vi "initializeArcus.vi"(1 "device_index (in) [0=def]":i32, 2 "read_timeout (ms); def=1000":i32=1000, 3 "write_timeout (ms); def=1000":i32=1000, 4 "clear_buffer? (T)":bool=TRUE, 5 "error in (no error)":errorcluster, 7 "error dialog? (T)":bool=TRUE) -> (14 "reference (out)":refnum<class "_Controller.lvclass">, 19 "error out":errorcluster)   [LabVIEW 2020, in "classes.lvlib" / "_Controller.lvclass"]
doc: "This VI establishes a reference to the USB Arcus controller at the specified index. Additionally, a LabVIEW based Class is instantiated, representing the specific device model. Additionally, parameters such as USB Reference, Index, Description, Name and other parameters are all set to the reference for ease of access downstream.\n\nOther inputs to be aware of:\n\n<B>device_index</B>: the index specific to the attached device (the index input is \"zero\" indexed - meaning the first of all devices sits at index = \"0\" and NOT \"1\")\n<B>read_timeout (ms)</B>: the USB \"read\" timeout in milliseconds (defaults to 1000ms)\n<B>write_timeout (ms)</B>: the USB \"write\" timeout in milliseconds (defaults to 1000ms)\n<B>clear_buffer?</B>: if set to TRUE, a USB Buffer CLEAR is issued (default is TRUE)\n<B>error_dialog?</B>: if set to TRUE, any errors triggered during USB controller communications result in a dialog window appearing at the moment the error is detected. If set to FALSE, the error is carried through via the error cluster. Default is TRUE.\n\nProduced By:\n\n<B>Kod Integrations, LLC</B>\n4835 Marianne Drive\nMount Airy, MD 21771\nhttp://www.kodintegrations.com\nemail: info@kodintegrations.com\nphone: (240) 687-1288"
uses:
  _Controller.lvclass
  DMXJSAController.lvclass
  Pmx4exSaController.lvclass
  ACESDEController.lvclass
  _SingleAxisController.lvclass
  PMX4CXSAController.lvclass
  PMX2EXSAController.lvclass
  C:/GEECS/Developers Version/source/Device Drivers/Newmark-NSC-A/Arcus Driver 3.0.0/ArcusUsbComm/classes/SingleAxisController/_SingleAxisController.lvclass
  C:/GEECS/Developers Version/source/Device Drivers/Newmark-NSC-A/Arcus Driver 3.0.0/ArcusUsbComm/classes/Controller/_Controller.lvclass
  C:/GEECS/Developers Version/source/Device Drivers/Newmark-NSC-A/Arcus Driver 3.0.0/ArcusUsbComm/classes/DMX-J-SA/DMXJSAController.lvclass
  C:/GEECS/Developers Version/source/Device Drivers/Newmark-NSC-A/Arcus Driver 3.0.0/ArcusUsbComm/classes/ACE-SDE/ACESDEController.lvclass
  C:/GEECS/Developers Version/source/Device Drivers/Newmark-NSC-A/Arcus Driver 3.0.0/ArcusUsbComm/classes/MultiAxisController/_MultiAxisController.lvclass
  C:/GEECS/Developers Version/source/Device Drivers/Newmark-NSC-A/Arcus Driver 3.0.0/ArcusUsbComm/classes/PMX-4EX-SA/Pmx4exSaController.lvclass
  C:/GEECS/Developers Version/source/Device Drivers/Newmark-NSC-A/Arcus Driver 3.0.0/ArcusUsbComm/classes/PMX-4CX-SA/PMX4CXSAController.lvclass
  C:/GEECS/Developers Version/source/Device Drivers/Newmark-NSC-A/Arcus Driver 3.0.0/ArcusUsbComm/classes/PMX-2EX-SA/PMX2EXSAController.lvclass
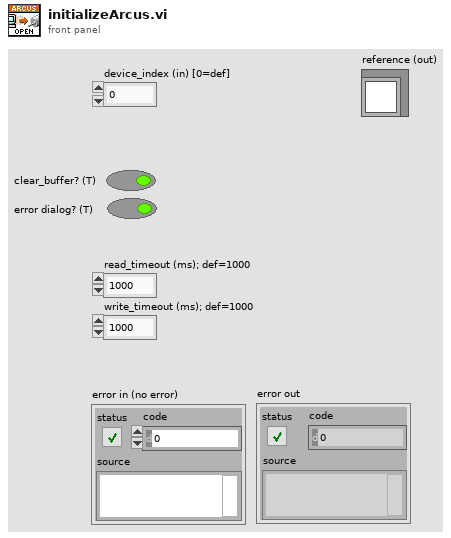
[diagram p1: front panel]
types:
  T1 = typedef "common.lvlib/device_info.ctl" = cluster{"device_name":string, "device_description":string, "model":T2}
  T2 = typedef "common.lvlib/models.ctl" = enum16{"<unrecognized>", "ACE-SDC", "ACE-SDE", "ACE-SXC", "ACE-SXE", "DMX-CAN", "DMX-J-SA", "DMX-K-SA", "DMX-UMD", "PMX-2ED-SA", "PMX-2EX-SA", "PMX-4CX-SA", "PMX-4EX-SA"}
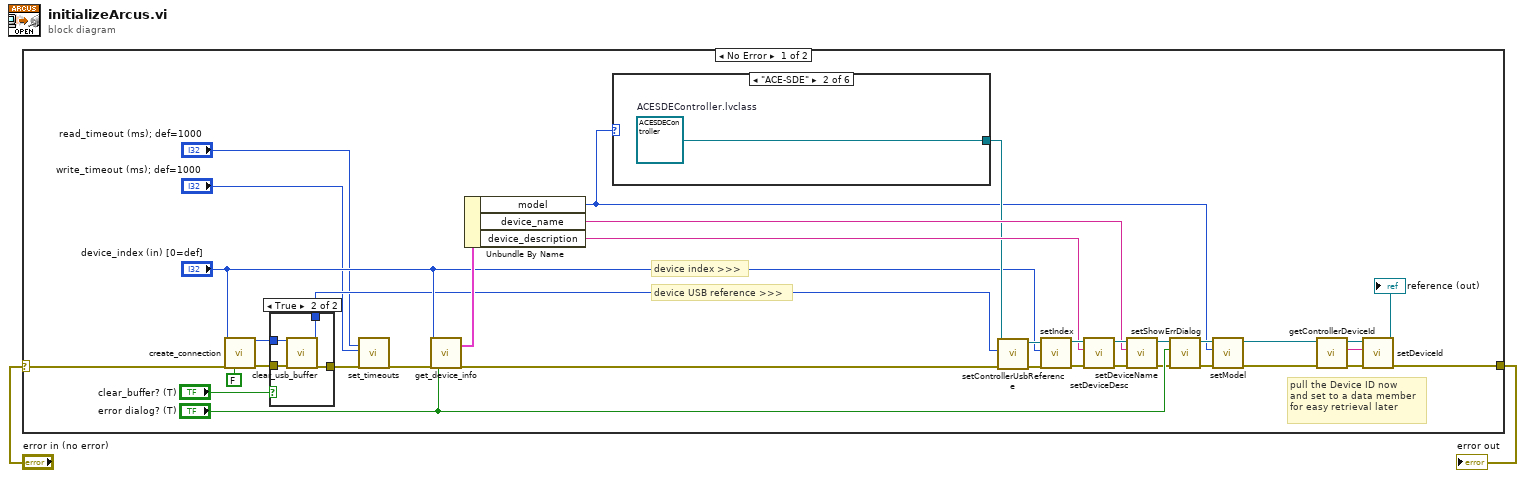
[diagram p0: block diagram]
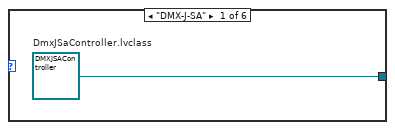
[diagram p3: hidden frame]
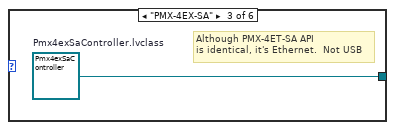
[diagram p4: hidden frame]
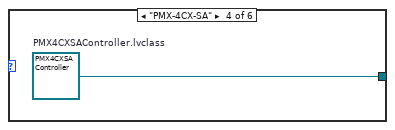
[diagram p5: hidden frame]
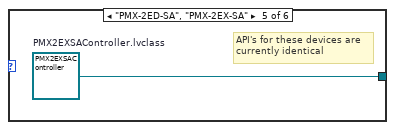
[diagram p6: hidden frame]
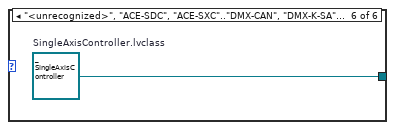
[diagram p7: hidden frame]
diagram:
  n1 = case shown="No Error" "error in (no error)" {
    selector: "error in (no error)" -> [w30 w50]
    tunnel: [w14 w50] -> w1
    frame No Error {
      # "device USB reference >>>"
      # "device index >>>"
      # "pull the Device ID now\nand set to a data member\nfor easy retrieval later"
      n2 = call "create_connection.vi"("device_index (def=0)"="device_index (in) [0=def]", "error in (no error)"=w30, "clear_buffer? (T)"=FALSE) -> ("reference"=w10:i32, "error out"=w8:errorcluster)  [unwired: 11 in]
      n3 = case shown="True" "clear_buffer? (T)" {
        tunnel: w10 -> [w39 w43]
        tunnel: [w39 w42] -> w9
        tunnel: w8 -> [w38 w41]
        tunnel: [w38 w40] -> w4
        frame False {
        }
        frame True {
          n4 = call "clear_usb_buffer.vi"("reference (in)"=w43, "error in (no error)"=w41) -> ("reference (out)"=w42:i32, "error out"=w40:errorcluster)  [unwired: 16 in]
        }
      }
      n5 = call "set_timeouts.vi"("read_timeout (ms); def=1000"="read_timeout (ms); def=1000", "write_timeout (ms); def=1000"="write_timeout (ms); def=1000", "error in (no error)"=w4) -> ("error out"=w3:errorcluster)  [unwired: 16 in]
      n6 = call "get_device_info.vi"("device_index (in)"="device_index (in) [0=def]", "error in (no error)"=w3, "dialog? (T)"="error dialog? (T)") -> ("device_info (out)"=w37:T1, "error out"=w29:errorcluster)  [unwired: 14 in, 1 out]
      n7 = Unbundle By Name(w37) -> ("model"=w20:T2, "device_name"=w31:string, "device_description"=w32:string)
      n8 = case shown="\"ACE-SDE\"" w20 {
        tunnel: [w44 w45 w46 w47 w48 w49] -> w27
        frame "DMX-J-SA" {
          w44 = refnum<class "DMXJSAController.lvclass"> refnum  # DmxJSaController.lvclass
        }
        frame "ACE-SDE" {
          w45 = refnum<class "ACESDEController.lvclass"> refnum  # ACESDEController.lvclass
        }
        frame "PMX-4EX-SA" {
          w46 = refnum<class "Pmx4exSaController.lvclass"> refnum  # Pmx4exSaController.lvclass
          # "Although PMX-4ET-SA API\nis identical, it's Ethernet.  Not USB"
        }
        frame "PMX-4CX-SA" {
          w47 = refnum<class "PMX4CXSAController.lvclass"> refnum  # PMX4CXSAController.lvclass
        }
        frame "PMX-2ED-SA", "PMX-2EX-SA" {
          w48 = refnum<class "PMX2EXSAController.lvclass"> refnum  # PMX2EXSAController.lvclass
          # "API's for these devices are\ncurrently identical"
        }
        frame "<unrecognized>", "ACE-SDC", "ACE-SXC".."DMX-CAN", "DMX-K-SA", "DMX-UMD" {
          w49 = refnum<class "_SingleAxisController.lvclass"> refnum  # SingleAxisController.lvclass
        }
      }
      n9 = call "setControllerUsbReference.vi"("error in (no error)"=w29, "reference"=w9, "reference (in)"=w27) -> ("error out"=w28:errorcluster, "reference (out)"=w26:refnum<class "_Controller.lvclass">)  [unwired: 7 in]
      n10 = call "setIndex.vi"("error in (no error)"=w28, "index"="device_index (in) [0=def]", "reference (in)"=w26) -> ("error out"=w36:errorcluster, "reference (out)"=w34:refnum<class "_Controller.lvclass">)  [unwired: 7 in]
      n11 = call "setDeviceDesc.vi"("error in (no error)"=w36, "deviceDesc"=w32, "reference (in)"=w34) -> ("error out"=w35:errorcluster, "reference (out)"=w33:refnum<class "_Controller.lvclass">)  [unwired: 7 in]
      n12 = call "setDeviceName.vi"("error in (no error)"=w35, "deviceName"=w31, "reference (in)"=w33) -> ("error out"=w23:errorcluster, "reference (out)"=w24:refnum<class "_Controller.lvclass">)  [unwired: 7 in]
      n13 = call "setShowErrDialog.vi"("error in (no error)"=w23, "showErrDialog"="error dialog? (T)", "reference (in)"=w24) -> ("error out"=w21:errorcluster, "reference (out)"=w22:refnum<class "_Controller.lvclass">)  [unwired: 7 in]
      n14 = call "setModel.vi"("error in (no error)"=w21, "model"=w20, "reference (in)"=w22) -> ("error out"=w19:errorcluster, "reference (out)"=w18:refnum<class "_Controller.lvclass">)  [unwired: 7 in]
      n15 = call "getControllerDeviceId.vi"("reference (in)"=w18, "error in (no error)"=w19) -> ("reference (out)"=w16:refnum<class "_Controller.lvclass">, "device_id (out)"=w17:string, "error out"=w15:errorcluster)  [unwired: 15 in]
      n16 = call "setDeviceId.vi"("error in (no error)"=w15, "deviceId"=w17, "reference (in)"=w16) -> ("error out"=w14:errorcluster, "reference (out)"=→"reference (out)":refnum<class "_Controller.lvclass">)  [unwired: 7 in]
    }
    frame Error {
    }
  }
  "error out" <- w1
